vi "3.4.vi"() -> ()   [LabVIEW 2017]
panel:
  in  "字符串 2":string
  in  "字符串":string
  out "结果字符串":string
  in  "输入 1":dbl
  in  "初始字符串":string
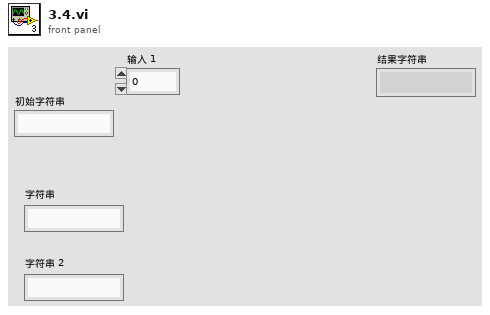
[diagram p1: front panel]
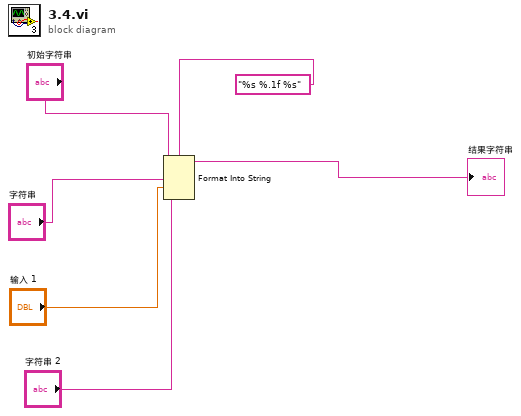
[diagram p0: block diagram]
diagram:
  n1 = Format Into String(format string="%s %.1f %s" ("格式字符串"), initial string="初始字符串", "字符串", "输入 1", "字符串 2") -> (resulting string=→"结果字符串":string)  [unwired: 1 in, 1 out]
